vi "DSF.Engine.BuilderManager.Initialize Builder Statuses.vi"(8 "error in (no error)":errorcluster, 11 "Builder Manager in":refnum<class "DSF.Engine.BuilderManager.lvclass">) -> (0 "error out":errorcluster, 2 "Builder Statuses":refnum<class "Status.Builder.lvclass">[](array[class]), 3 "Builder Manager out":refnum<class "DSF.Engine.BuilderManager.lvclass">)   [LabVIEW 2017, in "DSF.Engine.lvlib" / "DSF.Engine.BuilderManager.lvclass"]
uses:
  DSF.Engine.BuilderManager.lvclass
  Status/Status.Builder.lvclass
  DSF.Engine.BuilderManager.lvclass/DSF.Engine.BuilderManager.ctl
  <vilib>/National Instruments/Memory Manager/Classes/Pointer/Memory.Pointer.lvclass/Memory.Pointer.ctl
  <vilib>/National Instruments/Memory Manager/Classes/Pointer/Memory.Pointer.Parameter Check.Subset.vi
  <vilib>/National Instruments/Memory Manager/Classes/Pointer/Memory.Pointer.Get Address.vi
  <vilib>/National Instruments/Memory Manager/Classes/Pointer/Memory.Pointer.Encapsulate.vi
  <vilib>/National Instruments/Memory Manager/Classes/Pointer/Memory.Pointer.Parameter Check.Null Pointer.vi
  <vilib>/National Instruments/Memory Manager/Classes/Pointer/Memory.Pointer.Errors.vi
  <vilib>/National Instruments/Memory Manager/Classes/Pointer/Memory.Pointer.Errors.Out of Bounds.vi
  <vilib>/National Instruments/Memory Manager/Classes/Pointer/Memory.Pointer.Get Size.vi
  <vilib>/National Instruments/Memory Manager/Classes/Pointer/Memory.Pointer.Set Size.vi
  <vilib>/National Instruments/Memory Manager/Classes/Pointer/Memory.Pointer.Set Address.vi
  <vilib>/National Instruments/Memory Manager/Classes/Pointer/Memory.Pointer.Set Allocated.vi
  <vilib>/National Instruments/Memory Manager/Classes/Pointer/Memory.Pointer.Errors.Null Pointer.vi
  <vilib>/NI/Static Error Handling/VIs/Static Error Handling.Source Buffer.Write.String.vi
  <vilib>/National Instruments/Memory Manager/Classes/Pointer/Memory.Pointer.Errors.Write Pointer Size.vi
  <vilib>/National Instruments/Memory Manager/Classes/Pointer/Memory.Pointer.Errors.Create Error.vi
  <vilib>/NI/Static Error Handling/VIs/Static Error Handling.Source Buffer.Write.Numeric.Scalar.Base10.vi
  <vilib>/NI/Static Error Handling/VIs/Static Error Handling.Source Buffer.Write.Numeric.Scalar.Base10 (U64).vi
  <vilib>/NI/Static Error Handling/VIs/Static Error Handling.Error Cluster Constant.vi
  <vilib>/NI/Static Error Handling/VIs/Static Error Handling.Error Cluster Constant (512B).vi
  <vilib>/NI/Static Error Handling/VIs/Static Error Handling.Parameters.Status.Set.vi
  <vilib>/NI/Static Error Handling/VIs/Static Error Handling.Parameters.Code.Set.vi
  <vilib>/NI/Static Error Handling/VIs/Static Error Handling.Parameters.VI Source.Set.vi
  <vilib>/National Instruments/Memory Manager/Constants/Memory.Constants.vi
  <vilib>/National Instruments/Memory Manager/Constants/Memory.Constants.Library Name.vi
  <vilib>/National Instruments/Memory Manager/Classes/Pointer/Memory.Pointer.Errors.Get Info.vi
  Pointer/DSF.Engine.Pointer.Status.Builder.State.lvclass
  C:/Program Files (x86)/National Instruments/LabVIEW 2017/vi.lib/National Instruments/Memory Manager/Classes/Pointer/Memory.Pointer.lvclass
  <vilib>/National Instruments/Memory Manager/Classes/Pointer/Memory.Pointer.lvclass
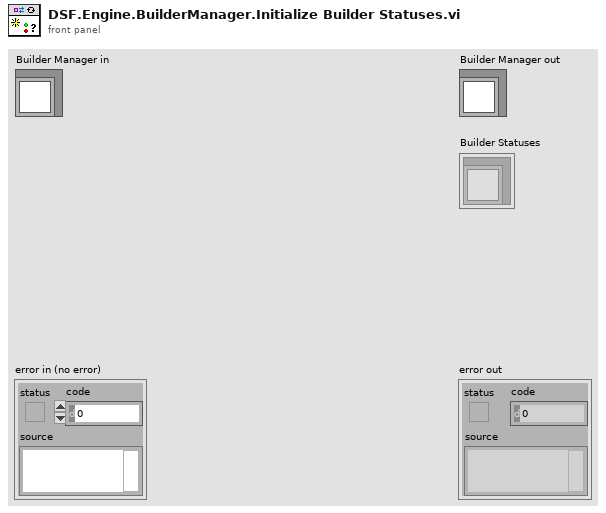
[diagram p1: front panel]
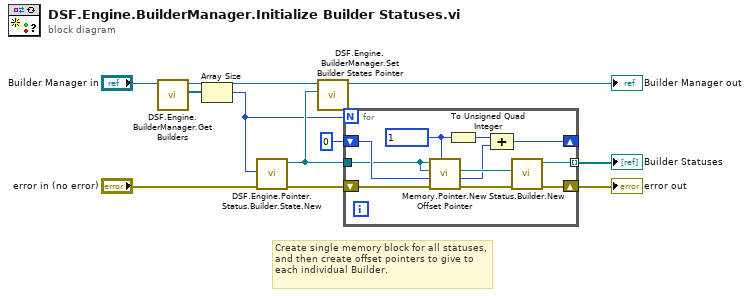
[diagram p0: block diagram]
diagram:
  # "Create single memory block for all statuses, and then create offset pointers to give to each individual Builder."
  n1 = call "DSF.Engine.BuilderManager.Get Builders.vi"("Builder Manager in"="Builder Manager in") -> ("Builders"=w2:refnum<class "DSF.Engine.Builder.lvclass">[], "Builder Manager out"=w3:refnum<class "DSF.Engine.BuilderManager.lvclass">)  [unwired: 9 in]
  n2 = Array Size(array=w2) -> (size(s)=w1:i32)
  n3 = call "DSF.Engine.Pointer.Status.Builder.State.New.vi"("error in (no error)"="error in (no error)", "count (1)"=w1) -> ("error out"=w8:errorcluster, "Builder State Pointer"=w5:refnum<class "DSF.Engine.Pointer.Status.Builder.State.lvclass">)  [unwired: 8 in]
  n4 = call "DSF.Engine.BuilderManager.Set Builder States Pointer.vi"("Builder States"=w5, "Builder Manager in"=w3) -> ("Builder Manager out"=→"Builder Manager out":refnum<class "DSF.Engine.BuilderManager.lvclass">)  [unwired: 9 in]
  n5 = for {
    N: w1 -> [_]
    shift-right: [w12] -> w6
    shift-left: w8 -> [w22]
    shift-right: [w21] -> _
    shift-left: u64 0 ("offset (0)") -> [w17]
    tunnel: w5 -> [w14]
    tunnel: [w13] -> w7 mode=indexing
    w20 = i64 1 ("length (-1: rest)")
    n6 = call <vilib>:"Memory.Pointer.New Offset Pointer.vi"("length (-1: rest)"=w20, "error in (no error)"=w22, "offset (0)"=w17, "offset Pointer type"=w14, "base Pointer in"=w14) -> ("error out"=w19:errorcluster, "offset out"=w15:u64, "offset Pointer"=w18:refnum<class "DSF.Engine.Pointer.Status.Builder.State.lvclass">)  [unwired: 3 in, 1 out]
    n7 = To Unsigned Quad Integer(1:w20) -> (0:w16:u64)
    n8 = Compound Arithmetic op=ADD(w16, w15) -> (w21:u64)
    n9 = call "Status.Builder.New.vi"("error in (no error)"=w19, "Builder State Pointer"=w18) -> ("error out"=w12:errorcluster, "Builder Status"=w13:refnum<class "Status.Builder.lvclass">)  [unwired: 8 in]
  }
  "error out" <- w6
  "Builder Statuses" <- w7
